vi "Configure Modulation Waveform Advanced (Dual-Sine).vi"(0 "VISA resource name":refnum<visa-resource-name>, 1 "Phase Offset (0 Rad)":dbl, 2 "Frequency (400 Hz)":dbl=400.0, 3 "Shape (0: Sine)":i32(ring) items=["Sine", "Triangle", "Square", "Ramp"], 5 "Modulation Type (0: Amplitude Modulation)":i32(ring) items=["Amplitude Modulation", "Frequency Modulation", "Phase Modulation", "Low Frequency Output"], 7 "Modulation Path (1: 1)":i32(ring)=1 items=["1"=1, "2"=2], 9 "Peak Percent (50)":dbl=50.0, 11 "error in (no error)":errorcluster, 12 "Tone Path (1: 1)":i32(ring)=1 items=["1"=1, "2"=2], 13 "Ramp Direction (0: Positive)":i32(ring) items=["Positive", "Negative"]) -> (4 "VISA resource name out":refnum<visa-resource-name>, 15 "error out":errorcluster)   [LabVIEW 2018, in "Agilent PSG MXG Series.lvlib"]
doc: "Configures the dual function generator source.\n\n<B>Notes:</B>\n1) This VI is valid only in N5171B, N5172B, N5181B, N5182B, N5173B, N5183B that install <B>Option UNT</B> and <B>Option 303</B> (AM, FM, phase modulation, and LF output)."
uses:
  Agilent PSG MXG Series.lvlib
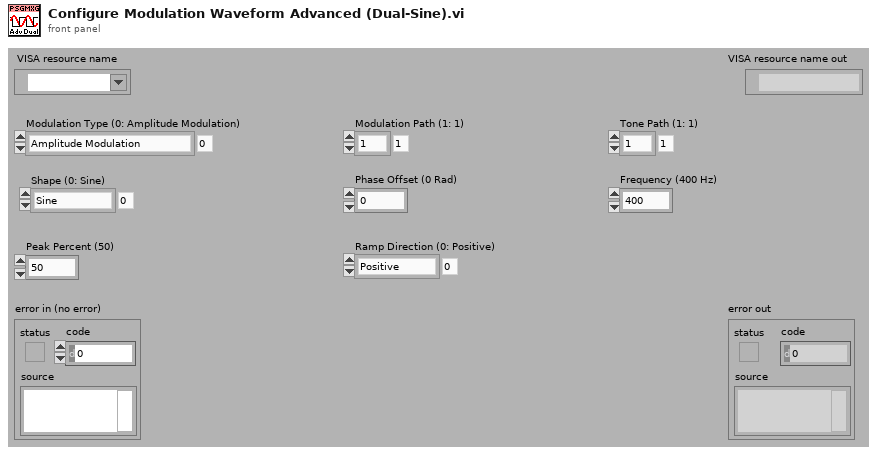
[diagram p1: front panel]
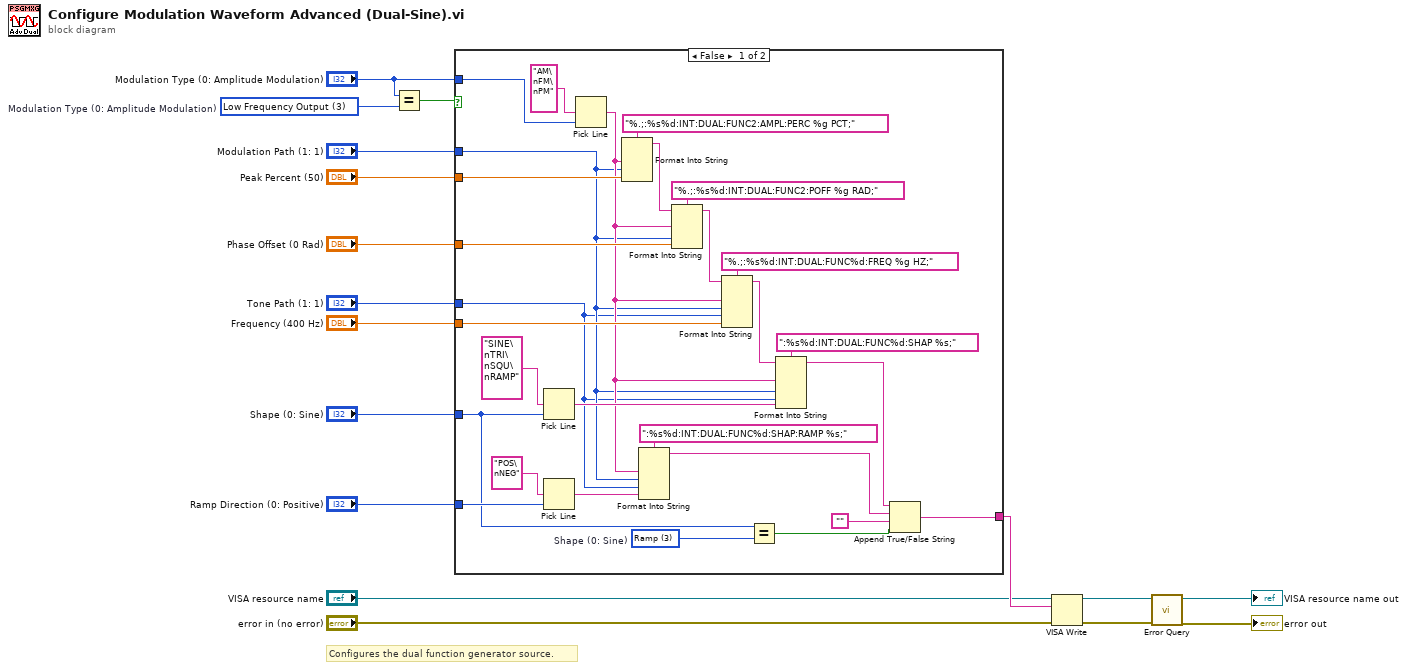
[diagram p0: block diagram]
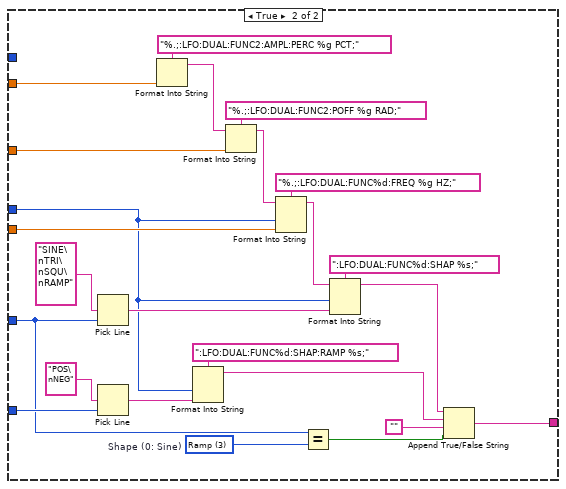
[diagram p2: hidden frame]
diagram:
  w8 = 3 items=["Amplitude Modulation", "Frequency Modulation", "Phase Modulation", "Low Frequency Output"]  # Modulation Type (0: Amplitude Modulation)
  # "Configures the dual function generator source."
  n1 = Equal?(x="Modulation Type (0: Amplitude Modulation)", y=w8) -> (x = y?=w7:bool)
  n2 = case shown="False" w7 {
    tunnel: "Shape (0: Sine)" -> [w20 w54]
    tunnel: "Ramp Direction (0: Positive)" -> [w36 w60]
    tunnel: [w18 w52] -> w15
    tunnel: "Modulation Type (0: Amplitude Modulation)" -> [w33 _]
    tunnel: "Modulation Path (1: 1)" -> [w27 _]
    tunnel: "Peak Percent (50)" -> [w32 w51]
    tunnel: "Phase Offset (0 Rad)" -> [w31 w50]
    tunnel: "Tone Path (1: 1)" -> [w26 w47]
    tunnel: "Frequency (400 Hz)" -> [w30 w49]
    frame False {
      w21 = 3 items=["Sine", "Triangle", "Square", "Ramp"]  # Shape (0: Sine)
      n3 = Pick Line(multi-line string="SINE\nTRI\nSQU\nRAMP", line index=w20) -> (output string=w29:string)  [unwired: 1 out]
      n4 = Pick Line(multi-line string="POS\nNEG", line index=w36) -> (output string=w25:string)  [unwired: 1 out]
      n5 = Pick Line(multi-line string="AM\nFM\nPM", line index=w33) -> (output string=w28:string)  [unwired: 1 out]
      n6 = Format Into String(format string="%.;:%s%d:INT:DUAL:FUNC2:AMPL:PERC %g PCT;", w28, w27, w32) -> (resulting string=w44:string)  [unwired: 2 in, 1 out]
      n7 = Format Into String(format string=":%s%d:INT:DUAL:FUNC%d:SHAP:RAMP %s;", w28, w27, w26, w25) -> (resulting string=w19:string)  [unwired: 2 in, 1 out]
      n8 = Format Into String(format string="%.;:%s%d:INT:DUAL:FUNC2:POFF %g RAD;", initial string=w44, w28, w27, w31) -> (resulting string=w42:string)  [unwired: 1 in, 1 out]
      n9 = Format Into String(format string="%.;:%s%d:INT:DUAL:FUNC%d:FREQ %g HZ;", initial string=w42, w28, w27, w26, w30) -> (resulting string=w39:string)  [unwired: 1 in, 1 out]
      n10 = Equal?(x=w20, y=w21) -> (x = y?=w22:bool)
      n11 = Format Into String(format string=":%s%d:INT:DUAL:FUNC%d:SHAP %s;", initial string=w39, w28, w27, w26, w29) -> (resulting string=w24:string)  [unwired: 1 in, 1 out]
      n12 = Append True/False String(1:w22, 2:"", 3:w19, 4:w24) -> (0:w18:string)
    }
    frame True {
      w55 = 3 items=["Sine", "Triangle", "Square", "Ramp"]  # Shape (0: Sine)
      n13 = Pick Line(multi-line string="SINE\nTRI\nSQU\nRAMP", line index=w54) -> (output string=w48:string)  [unwired: 1 out]
      n14 = Pick Line(multi-line string="POS\nNEG", line index=w60) -> (output string=w46:string)  [unwired: 1 out]
      n15 = Format Into String(format string="%.;:LFO:DUAL:FUNC2:AMPL:PERC %g PCT;", w51) -> (resulting string=w68:string)  [unwired: 2 in, 1 out]
      n16 = Format Into String(format string=":LFO:DUAL:FUNC%d:SHAP:RAMP %s;", w47, w46) -> (resulting string=w53:string)  [unwired: 2 in, 1 out]
      n17 = Format Into String(format string="%.;:LFO:DUAL:FUNC2:POFF %g RAD;", initial string=w68, w50) -> (resulting string=w66:string)  [unwired: 1 in, 1 out]
      n18 = Format Into String(format string="%.;:LFO:DUAL:FUNC%d:FREQ %g HZ;", initial string=w66, w47, w49) -> (resulting string=w63:string)  [unwired: 1 in, 1 out]
      n19 = Equal?(x=w54, y=w55) -> (x = y?=w56:bool)
      n20 = Format Into String(format string=":LFO:DUAL:FUNC%d:SHAP %s;", initial string=w63, w47, w48) -> (resulting string=w58:string)  [unwired: 1 in, 1 out]
      n21 = Append True/False String(1:w56, 2:"", 3:w53, 4:w58) -> (0:w52:string)
    }
  }
  n22 = VISA Write(VISA resource name="VISA resource name", write buffer=w15, error in (no error)="error in (no error)") -> (VISA resource name out=w12:refnum<visa-resource-name>, error out=w11:errorcluster)  [unwired: 1 out]
  n23 = call "Error Query.vi"("error in (no error)"=w11, "VISA resource name"=w12) -> ("error out"=→"error out":errorcluster, "VISA resource name out"=→"VISA resource name out":refnum<visa-resource-name>)  [unwired: 8 out]
